vi "LDA Control.vi"() -> (1 "Error":errorcluster)   [LabVIEW 2022 SP3]
uses:
  File/Setup_Filetype.ctl
  Globals/LDA_global.vi
panel:
  out "Allowable":bool[](array[boolean])=[TRUE, TRUE, FALSE, FALSE, FALSE, TRUE, FALSE, FALSE, FALSE, FALSE, FALSE, FALSE]
  in  "Mode":i32(listbox)
  out "BSA IP Number":string
  out "Setup String":string
  out "Setup Filename":string
  out "reference out":refnum<k7>
  in  "SysMon":refnum<k7>(container)
  in  "Set Power (mW)":dbl=150.0
  in  "Laser":i32[](listbox)
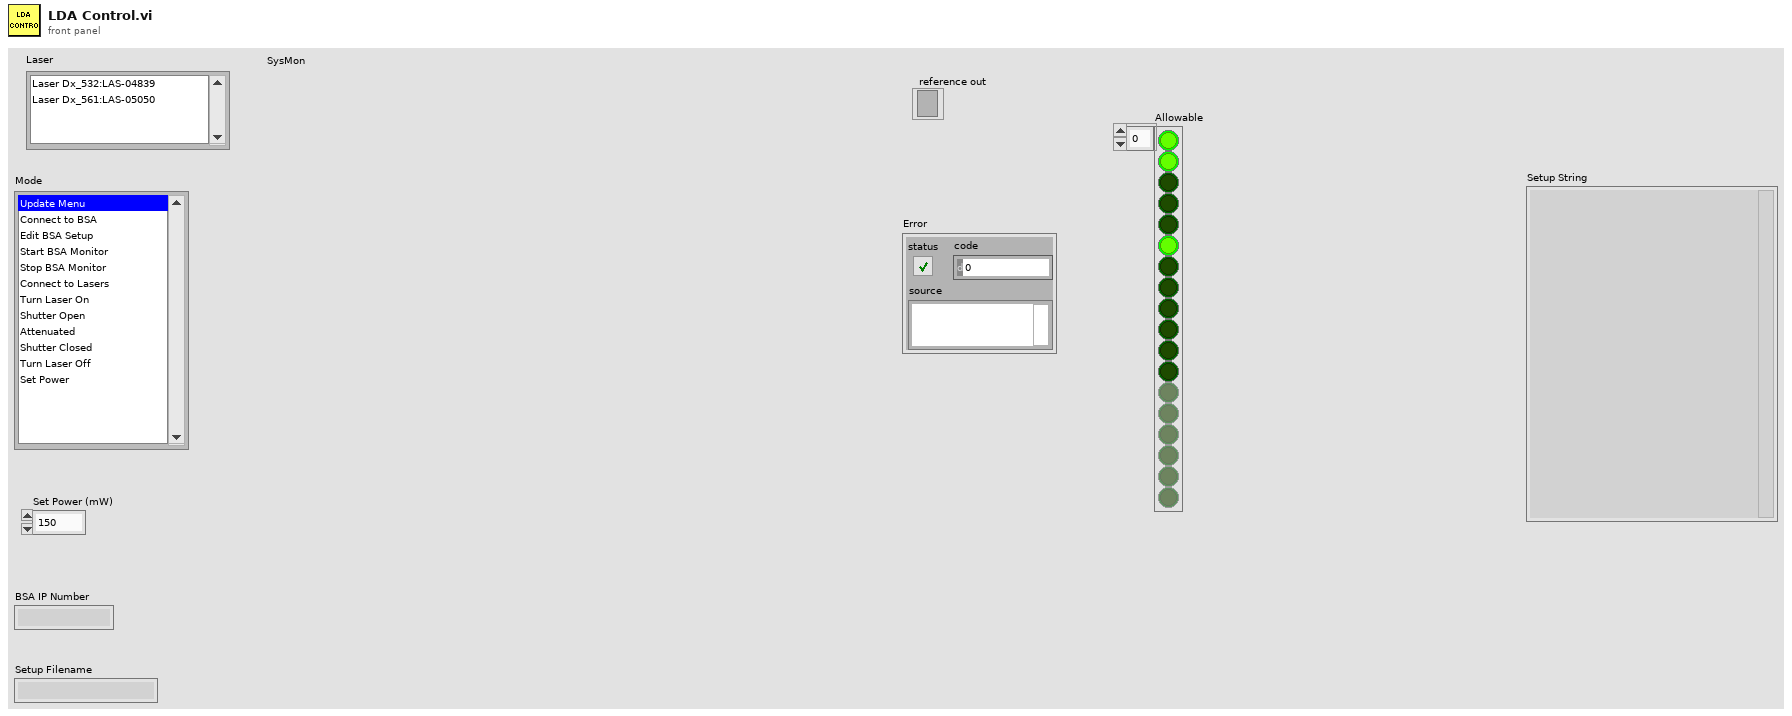
[diagram p1: front panel]
types:
  T1 = enum16{"Zero or one", "One", "Zero or more", "One or more"}
  T2 = typedef "Setup_Filetype.ctl" = enum16{"Measurement Setups", "Calibration Setups", "General", "Results File Plotter Setups", "Speed Calib Tweaks"}
  T3 = typedef "LDA_Channel.ctl" = cluster{"Wavelength (nm)":dbl, "Vel Comp":string, "Max Velocity":dbl, "Min Velocity":dbl, "Max Record length":u16, "Signal gain (dB)":i16, "High voltage":i16, "Optics Conversion Factor":dbl, "Min Record length":u16, "Multiply Velocity by -1":bool, "Signal to Noise Ratio":string, "Validation Ratio":string, "Probe":string, "Laser":string, "BSA":string, "Lense":string, "Beam Separation (mm)":dbl, "Focal Length (mm)":dbl, "COLOUR":u32, "BSA IP":string, "Velocity Range (m/s)":dbl, "Centre Velocity (m/s)":dbl, "Unshifted mW":dbl, "Shifted mW":dbl, "Bandwidth Hz":dbl, "Req Sampling Rate Hz":dbl, "Ch":i32, "CenterFreq Hz":dbl, "Laser IP":string, "Sync Delay (s)":dbl}
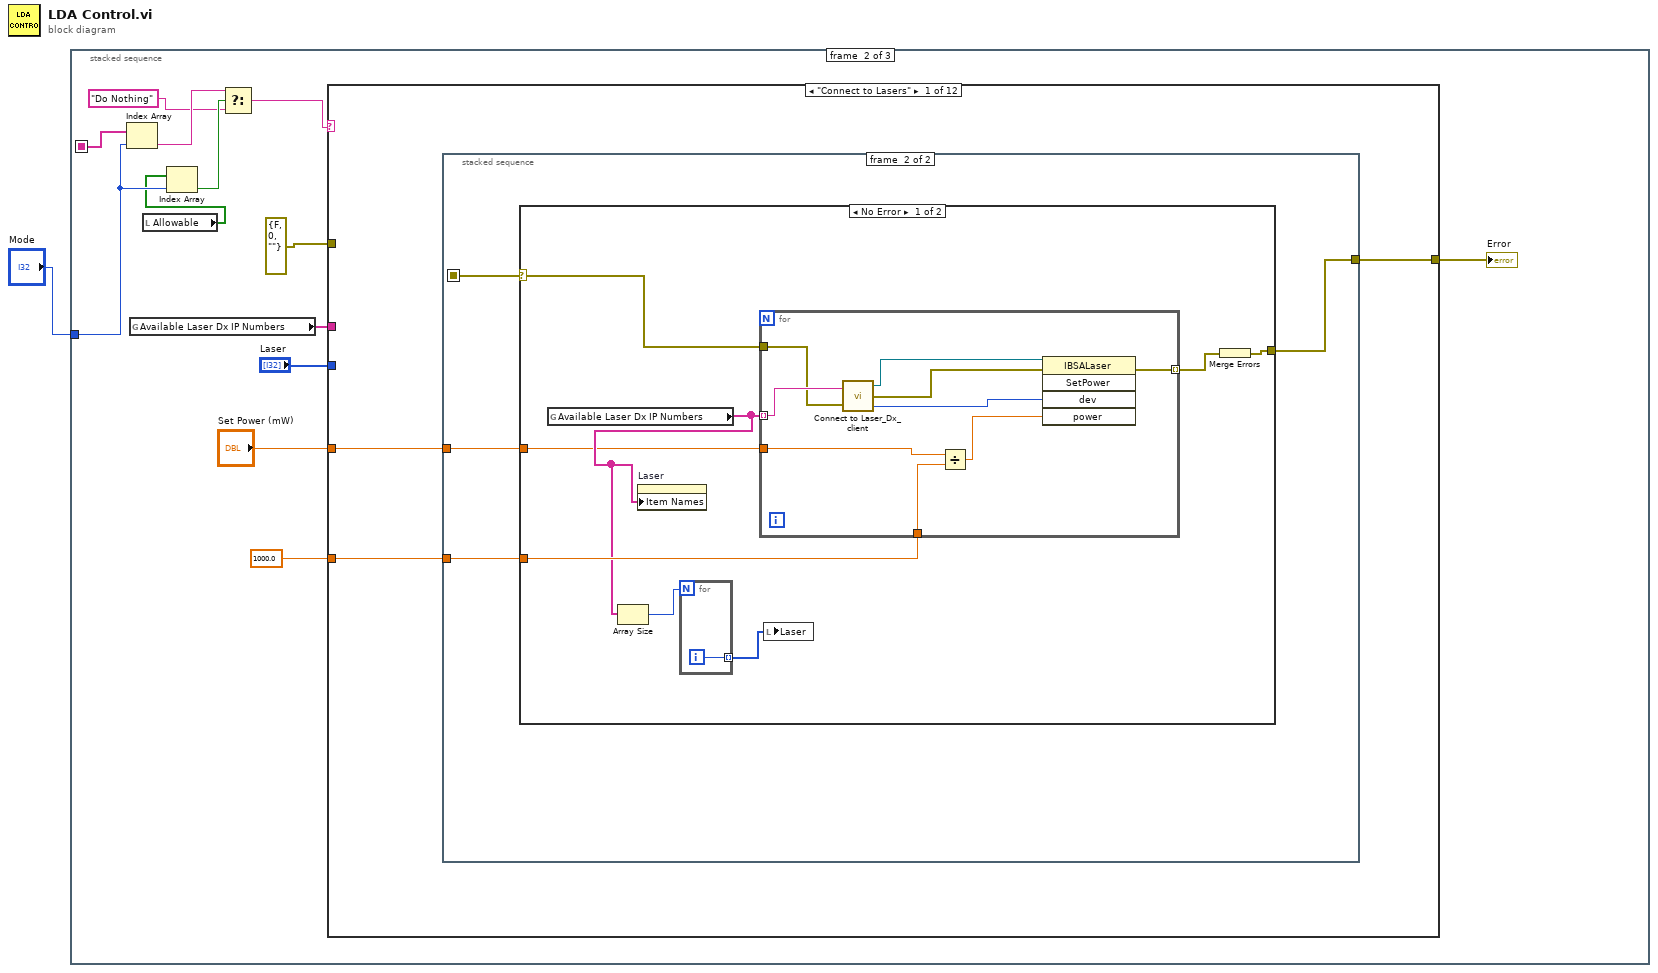
[diagram p0: block diagram]
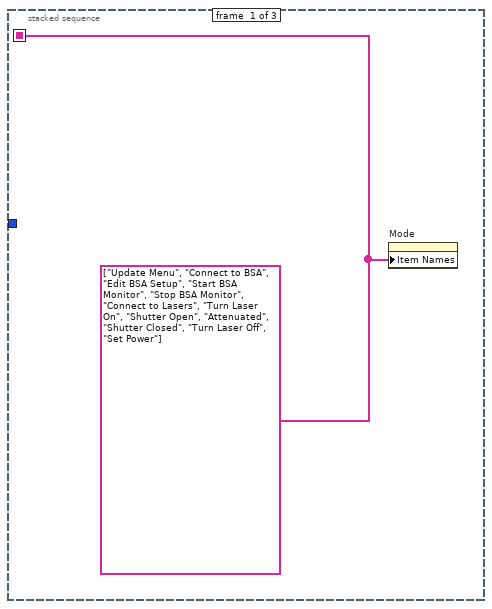
[diagram p2: hidden frame]
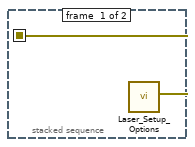
[diagram p3: hidden frame]
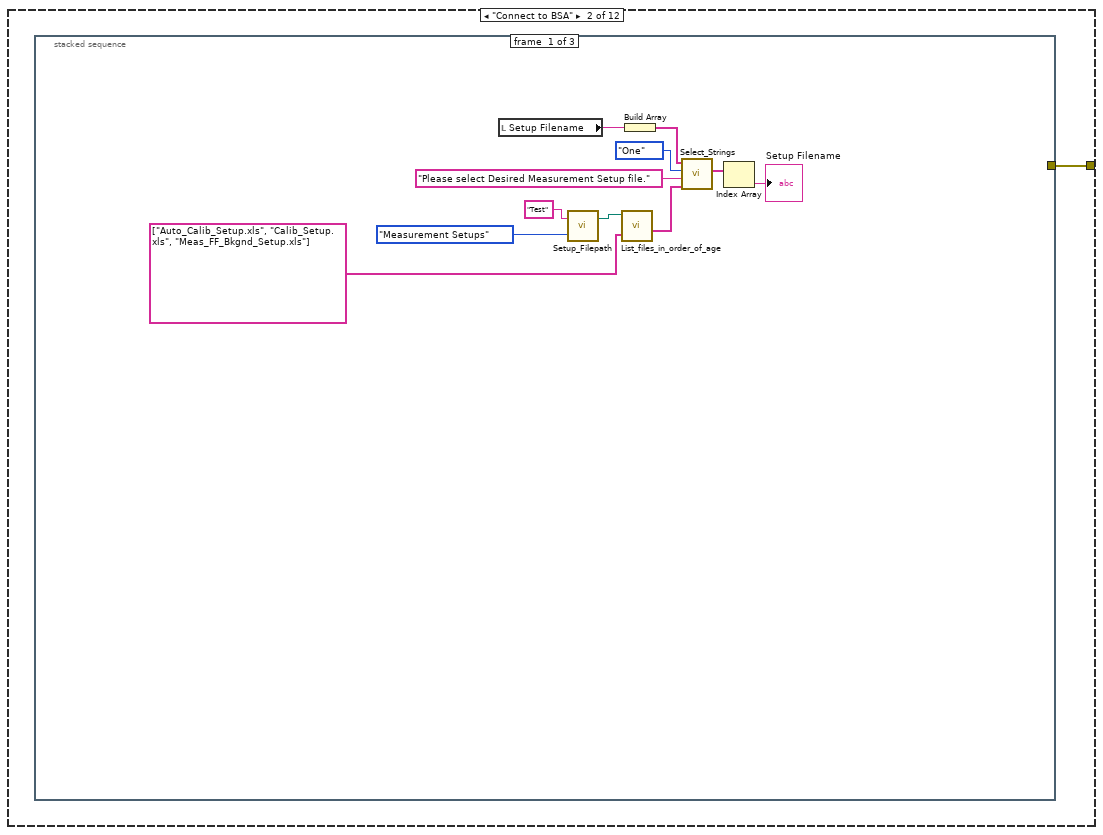
[diagram p5: hidden frame]
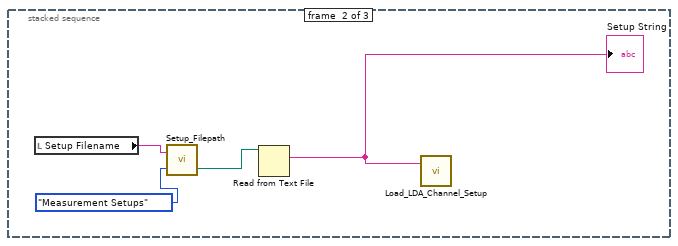
[diagram p6: hidden frame]
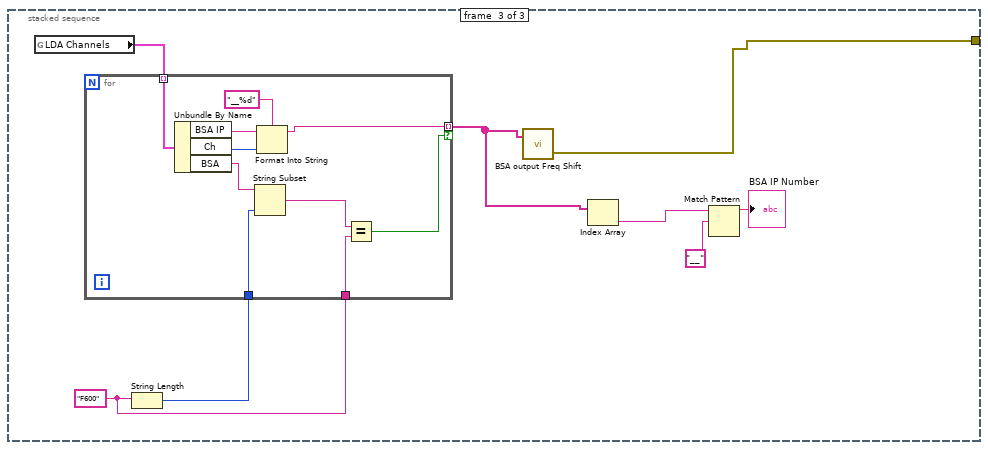
[diagram p7: hidden frame]
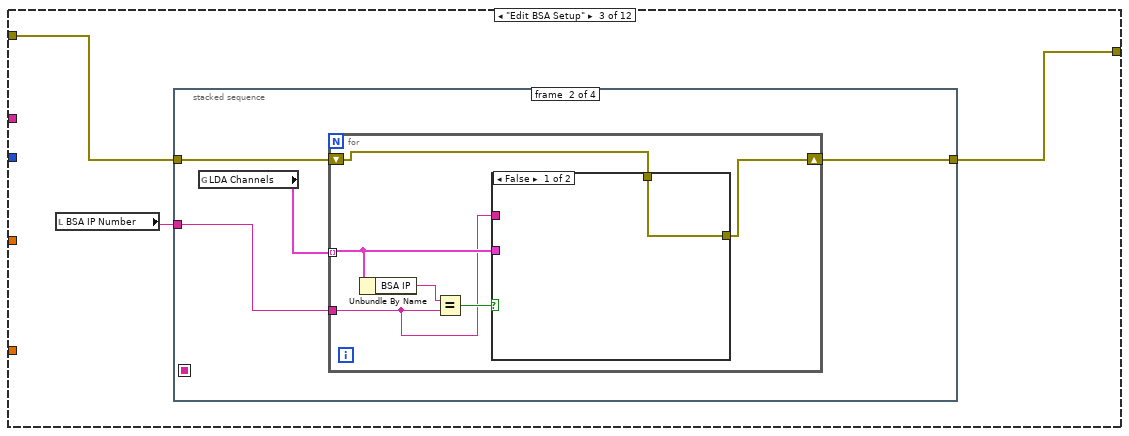
[diagram p8: hidden frame]
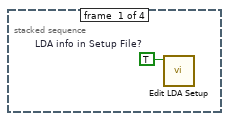
[diagram p9: hidden frame]
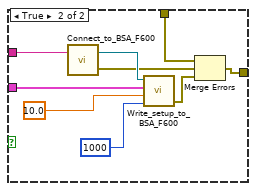
[diagram p10: hidden frame]
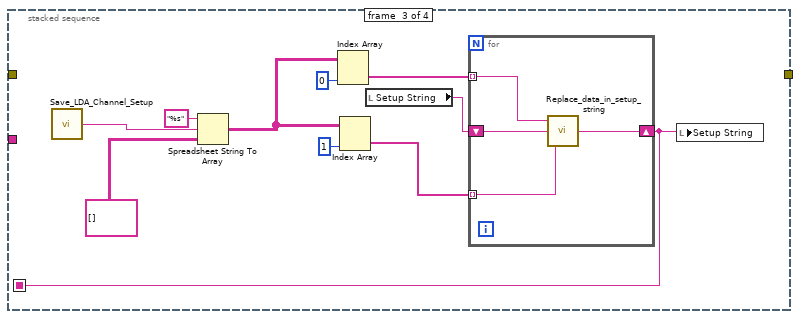
[diagram p11: hidden frame]
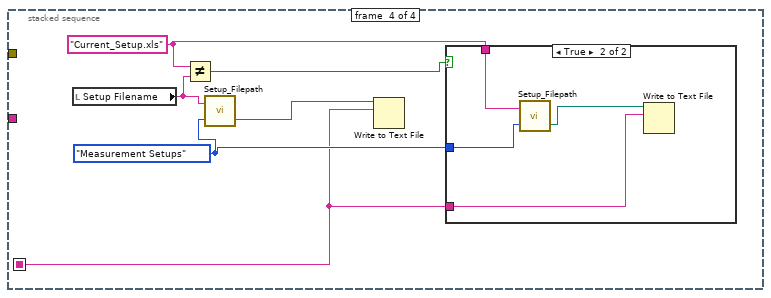
[diagram p12: hidden frame]
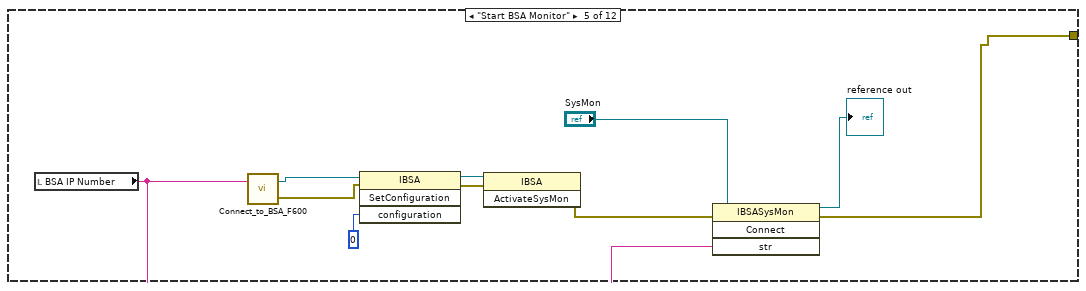
[diagram p15: hidden frame]
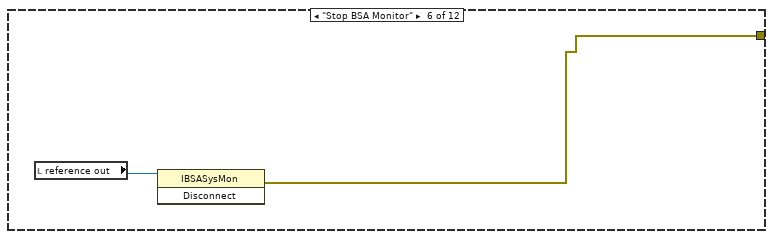
[diagram p16: hidden frame]
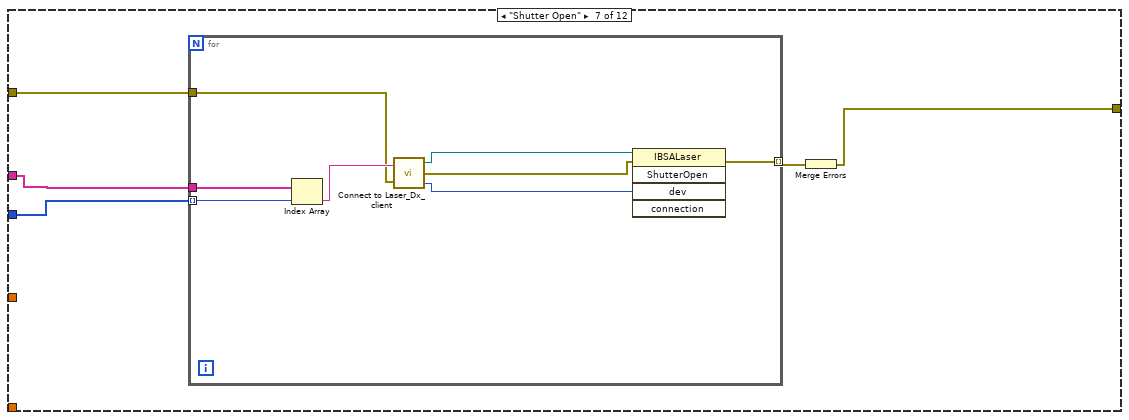
[diagram p17: hidden frame]
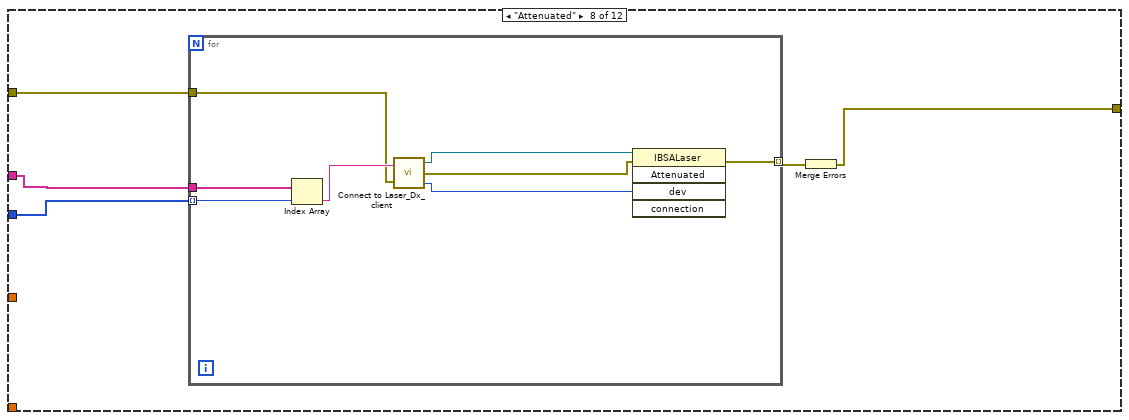
[diagram p18: hidden frame]
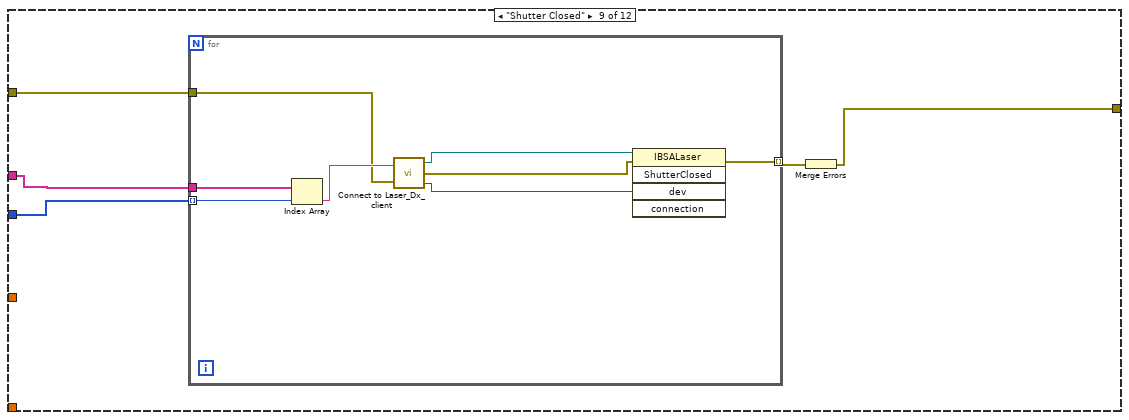
[diagram p19: hidden frame]
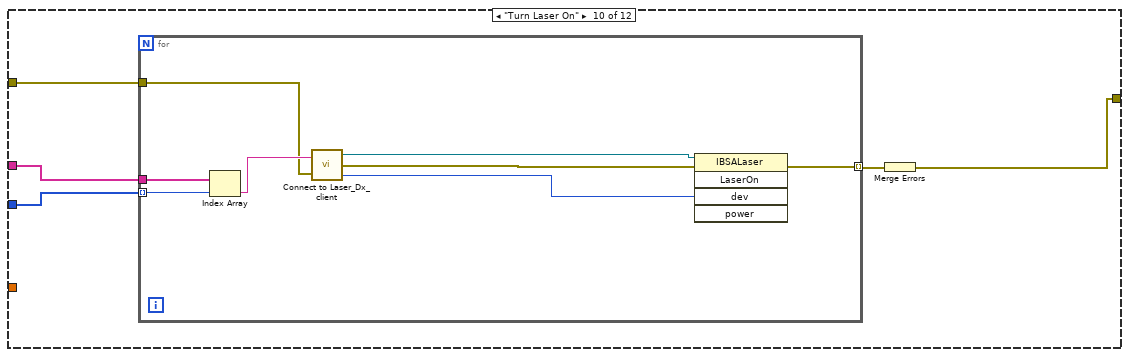
[diagram p20: hidden frame]
diagram:
  n1 = stacked-sequence {
    seq-local: [w2 _ _] -> [_ w11 _]
    tunnel: "Mode" -> [_ w8 _]
    frame #0 {
      w2 = string[] ["Update Menu", "Connect to BSA", "Edit BSA Setup", "Start BSA Monitor", "Stop BSA Monitor", "Connect to Lasers", "Turn Laser On", "Shutter Open", "Attenuated", "Shutter Closed", "Turn Laser Off", "Set Power"] ("Item Names")
      n2 = property on="Mode" class="LstBox (strict)"("Item Names"=w2) -> ()  [unwired: 2 in, 2 out]
    }
    frame #1 {
      n3 = Index Array(array=w11, index=w8) -> (element=w5:string)
      n4 = global read "LDA_global.vi" "Available Laser Dx IP Numbers"() -> (w13:string[])
      n5 = local read "Allowable"() -> (w7:bool[])
      n6 = Index Array(array=w7, index=w8) -> (element=w6:bool)
      n7 = Select(t=w5, s=w6, f="Do Nothing" ("t")) -> (s? t:f=w10:string)
      n8 = case shown="\"Connect to Lasers\"" w10 {
        tunnel: [w17 w43 w78 w125 w126 w136 w139 w152 w165 w178 w191 w205] -> w12
        tunnel: 1000.0 ("y") -> [w18 _ _ _ _ _ _ _ _ _ _ w209]
        tunnel: "Laser" -> [_ _ _ _ _ _ w141 w154 w167 w180 w193 w207]
        tunnel: w13 -> [_ _ _ _ _ _ w142 w155 w168 w181 w194 w208]
        tunnel: errorcluster {"status"=FALSE, "code"=0, "source"=""} ("error IO") -> [_ _ w77 w125 _ _ w138 w151 w164 w177 w190 w204]
        tunnel: "Set Power (mW)" -> [w16 _ _ _ _ _ _ _ _ _ _ w203]
        frame "Connect to Lasers" {
          n9 = stacked-sequence {
            seq-local: [w19 _] -> [_ w21]
            tunnel: w18 -> [_ w23]
            tunnel: [_ w22] -> w17
            tunnel: w16 -> [_ w20]
            frame #0 {
              n10 = call "Laser_Setup_Options.vi"() -> ("error out"=w19:errorcluster)  [unwired: 5 in, 3 out]
            }
            frame #1 {
              n11 = case shown="No Error" w21 {
                selector: w21 -> [w30 w42]
                tunnel: w23 -> [w31 _]
                tunnel: [w28 w42] -> w22
                tunnel: w20 -> [w24 _]
                frame No Error {
                  n12 = global read "LDA_global.vi" "Available Laser Dx IP Numbers"() -> (w27:string[])
                  n13 = Array Size(array=w27) -> (size(s)=w25:i32)
                  n14 = property on="Laser" class="LstBox (strict)"("Item Names"=w27) -> ()  [unwired: 2 in, 2 out]
                  n15 = for {
                    N: w25 -> [_]
                    tunnel: [w32] -> w26 mode=indexing
                    i -> [w32]
                  }
                  n16 = for {
                    tunnel: w27 -> [w36] mode=indexing
                    tunnel: w31 -> [w41]
                    tunnel: w30 -> [w35]
                    tunnel: [w34] -> w29 mode=indexing
                    tunnel: w24 -> [w33]
                    n17 = call "Connect to Laser_Dx_client.vi"("Laser IP Number"=w36, "error in (no error)"=w35) -> ("Laser_Dx"=w39:refnum<k7>, "error out"=w38:errorcluster, "Channel"=w37:i64)
                    n18 = Divide(x=w33, y=w41) -> (x/y=w40:dbl)
                    n19 = invoke class="IBSALaser" method="SetPower"(reference=w39, error in=w38, "dev"=w37, "power"=w40) -> (error out=w34:errorcluster)  [unwired: 1 in, 4 out]
                  }
                  n20 = local write "Laser"(w26) -> ()
                  n21 = Merge Errors(w29) -> (w28:errorcluster)
                }
                frame Error {
                }
              }
            }
          }
        }
        frame "Connect to BSA" {
          n22 = stacked-sequence {
            tunnel: [_ _ w65] -> w43
            frame #0 {
              n23 = local read "Setup Filename"() -> (w52:string)
              n24 = call "Setup_Filepath.vi"("Setup File Type"=Setup_Filetype."Measurement Setups", "Filename in"="Test") -> ("Directory"=w49:path)  [unwired: 1 out]
              n25 = call "List_files_in_order_of_age.vi"("Files to Hide"=string[] ["Auto_Calib_Setup.xls", "Calib_Setup.xls", "Meas_FF_Bkgnd_Setup.xls"] ("file names"), "Folder"=w49) -> ("file names"=w50:string[])  [unwired: 9 in]
              n26 = Build Array(w52) -> (w53:string[])
              n27 = call "Select_Strings.vi"("Available Ch names"=w50, "Message"="Please select Desired Measurement Setup file.", "Selector mode"=T1."One", "Desired Ch names (in)"=w53) -> ("Selected Channel Names"=w51:string[])  [unwired: 2 in, 2 out]
              n28 = Index Array(array=w51) -> (element=→"Setup Filename":string)  [unwired: 1 in]
            }
            frame #1 {
              n29 = local read "Setup Filename"() -> (w58:string)
              n30 = call "Setup_Filepath.vi"("Setup File Type"=Setup_Filetype."Measurement Setups", "Filename in"=w58) -> ("Filename Out"=w56:path)  [unwired: 1 out]
              n31 = Read from Text File(file (use dialog)=w56) -> (text=w57:string)  [unwired: 3 in, 3 out]
              "Setup String" <- w57
              n32 = call "Load_LDA_Channel_Setup.vi"("Setup file string"=w57) -> ()  [unwired: 2 in]
            }
            frame #2 {
              w59 = "F600"
              n33 = global read "LDA_global.vi" "LDA Channels"() -> (w66:T3[])
              n34 = String Length(string=w59) -> (length=w60:i32)
              n35 = for {
                tunnel: [w72] -> w62 mode=indexing if=w67
                tunnel: w66 -> [w76] mode=indexing
                tunnel: w60 -> [w70]
                tunnel: w59 -> [w68]
                n36 = Unbundle By Name(w76) -> ("BSA IP"=w74:string, "Ch"=w75:i32, "BSA"=w71:string)
                n37 = String Subset(string=w71, length (rest)=w70) -> (substring=w69:string)  [unwired: 1 in]
                n38 = Format Into String(format string="__%d", initial string=w74, w75) -> (resulting string=w72:string)  [unwired: 1 in, 1 out]
                n39 = Equal?(x=w69, y=w68) -> (x = y?=w67:bool)
              }
              n40 = call "BSA output Freq Shift.vi"("BSAIP__ChNum"=w62) -> ("BSA Error"=w65:errorcluster)  [unwired: 2 in]
              n41 = Index Array(array=w62) -> (element=w64:string)  [unwired: 1 in]
              n42 = Match Pattern(string=w64, regular expression="__" ("string")) -> (before substring=→"BSA IP Number":string)  [unwired: 1 in, 3 out]
            }
          }
        }
        frame "Edit BSA Setup" {
          n43 = local read "BSA IP Number"() -> (w79:string)
          n44 = stacked-sequence {
            seq-local: [_ _ w101 _] -> [_ _ _ w115]
            tunnel: w79 -> [_ w83 _ _]
            tunnel: [_ w82 _ _] -> w78
            tunnel: w77 -> [_ w81 _ _]
            frame #0 {
              w80 = TRUE  # LDA info in Setup File?
              n45 = call "Edit LDA Setup.vi"("LDA info in Setup File?"=w80) -> ()  [unwired: 11 in]
            }
            frame #1 {
              n46 = global read "LDA_global.vi" "LDA Channels"() -> (w84:T3[])
              n47 = for {
                tunnel: w84 -> [w90] mode=indexing
                tunnel: w83 -> [w87]
                shift-right: [w85] -> w82
                shift-left: w81 -> [w86]
                n48 = Unbundle By Name(w90) -> ("BSA IP"=w89:string)
                n49 = Equal?(x=w89, y=w87) -> (x = y?=w88:bool)
                n50 = case shown="False" w88 {
                  tunnel: w90 -> [_ w98]
                  tunnel: w87 -> [_ w97]
                  tunnel: [w91 w93] -> w85
                  tunnel: w86 -> [w91 w92]
                  frame False {
                  }
                  frame True {
                    n51 = call "Connect_to_BSA_F600.vi"("BSA IP Number"=w97) -> ("error out"=w94:errorcluster, "F600"=w96:refnum<k7>)  [unwired: 1 in]
                    n52 = call "Write_setup_to_BSA_F600.vi"("No Of Samples"=1000, "Time (s)"=sgl 10.0, "BSA Setup In"=w98, "BSACtrl.IBSA F600"=w96) -> ("error out"=w95:errorcluster)  [unwired: 2 out]
                    n53 = Merge Errors(w92, w94, w95) -> (w93:errorcluster)
                  }
                }
              }
            }
            frame #2 {
              n54 = call "Save_LDA_Channel_Setup.vi"() -> ("Setup file string"=w110:string)  [unwired: 1 in]
              n55 = Spreadsheet String To Array(format string="%s", spreadsheet string=w110, array type (2D Dbl)=string[][] []) -> (array=w109:string[][])  [unwired: 1 in]
              n56 = Index Array(array=w109, index (col)=0 ("disabled index (col)")) -> (element=w108:string[])  [unwired: 1 in]
              n57 = Index Array(array=w109, index (col)=1 ("disabled index (col)")) -> (element=w107:string[])  [unwired: 1 in]
              n58 = local read "Setup String"() -> (w106:string)
              n59 = for {
                tunnel: w108 -> [w114] mode=indexing
                tunnel: w107 -> [w112] mode=indexing
                shift-right: [w111] -> w101
                shift-left: w106 -> [w113]
                n60 = call "Replace_data_in_setup_string.vi"("New data string"=w112, "Input string"=w113, "Variable name"=w114) -> ("Appended string"=w111:string)
              }
              n61 = local write "Setup String"(w101) -> ()
            }
            frame #3 {
              w117 = "Current_Setup.xls"
              w116 = Setup_Filetype."Measurement Setups" ("Setup File Type")
              n62 = local read "Setup Filename"() -> (w119:string)
              n63 = Not Equal?(x=w117, y=w119) -> (x != y?=w118:bool)
              n64 = call "Setup_Filepath.vi"("Setup File Type"=w116, "Filename in"=w119) -> ("Filename Out"=w120:path)  [unwired: 1 out]
              n65 = Write to Text File(file (use dialog)=w120, text=w115) -> ()  [unwired: 2 in, 3 out]
              n66 = case shown="True" w118 {
                tunnel: w117 -> [_ w124]
                tunnel: w116 -> [_ w123]
                tunnel: w115 -> [_ w122]
                frame False {
                }
                frame True {
                  n67 = call "Setup_Filepath.vi"("Setup File Type"=w123, "Filename in"=w124) -> ("Filename Out"=w121:path)  [unwired: 1 out]
                  n68 = Write to Text File(file (use dialog)=w121, text=w122) -> ()  [unwired: 2 in, 3 out]
                }
              }
            }
          }
        }
        frame "Do Nothing", Default {
        }
        frame "Start BSA Monitor" {
          n69 = local read "BSA IP Number"() -> (w127:string)
          n70 = call "Connect_to_BSA_F600.vi"("BSA IP Number"=w127) -> ("error out"=w135:errorcluster, "F600"=w134:refnum<k7>)  [unwired: 1 in]
          n71 = invoke class="IBSA" method="SetConfiguration"(reference=w134, error in=w135, "configuration"=0 ("config")) -> (reference out=w130:refnum<k7>, error out=w129:errorcluster)  [unwired: 1 in, 2 out]
          n72 = invoke class="IBSA" method="ActivateSysMon"(reference=w130, error in=w129) -> (error out=w131:errorcluster)  [unwired: 1 in, 2 out]
          n73 = invoke class="IBSASysMon" method="Connect"(reference="SysMon", error in=w131, "str"=w127) -> (reference out=→"reference out":refnum<k7>, error out=w126:errorcluster)  [unwired: 1 in, 2 out]
        }
        frame "Stop BSA Monitor" {
          n74 = local read "reference out"() -> (w137:refnum<k7>)
          n75 = invoke class="IBSASysMon" method="Disconnect"(reference=w137) -> (error out=w136:errorcluster)  [unwired: 2 in, 2 out]
        }
        frame "Shutter Open" {
          n76 = for {
            tunnel: [w150] -> w140 mode=indexing
            tunnel: w142 -> [w148]
            tunnel: w141 -> [w147] mode=indexing
            tunnel: w138 -> [w143]
            n77 = Index Array(array=w148, index=w147) -> (element=w149:string)
            n78 = call "Connect to Laser_Dx_client.vi"("Laser IP Number"=w149, "error in (no error)"=w143) -> ("Laser_Dx"=w146:refnum<k7>, "error out"=w145:errorcluster, "Channel"=w144:i64)
            n79 = invoke class="IBSALaser" method="ShutterOpen"(reference=w146, error in=w145, "dev"=w144) -> (error out=w150:errorcluster)  [unwired: 2 in, 4 out]
          }
          n80 = Merge Errors(w140) -> (w139:errorcluster)
        }
        frame "Attenuated" {
          n81 = for {
            tunnel: [w163] -> w153 mode=indexing
            tunnel: w155 -> [w161]
            tunnel: w154 -> [w160] mode=indexing
            tunnel: w151 -> [w156]
            n82 = Index Array(array=w161, index=w160) -> (element=w162:string)
            n83 = call "Connect to Laser_Dx_client.vi"("Laser IP Number"=w162, "error in (no error)"=w156) -> ("Laser_Dx"=w159:refnum<k7>, "error out"=w158:errorcluster, "Channel"=w157:i64)
            n84 = invoke class="IBSALaser" method="Attenuated"(reference=w159, error in=w158, "dev"=w157) -> (error out=w163:errorcluster)  [unwired: 2 in, 4 out]
          }
          n85 = Merge Errors(w153) -> (w152:errorcluster)
        }
        frame "Shutter Closed" {
          n86 = for {
            tunnel: [w176] -> w166 mode=indexing
            tunnel: w168 -> [w174]
            tunnel: w167 -> [w173] mode=indexing
            tunnel: w164 -> [w169]
            n87 = Index Array(array=w174, index=w173) -> (element=w175:string)
            n88 = call "Connect to Laser_Dx_client.vi"("Laser IP Number"=w175, "error in (no error)"=w169) -> ("Laser_Dx"=w172:refnum<k7>, "error out"=w171:errorcluster, "Channel"=w170:i64)
            n89 = invoke class="IBSALaser" method="ShutterClosed"(reference=w172, error in=w171, "dev"=w170) -> (error out=w176:errorcluster)  [unwired: 2 in, 4 out]
          }
          n90 = Merge Errors(w166) -> (w165:errorcluster)
        }
        frame "Turn Laser On" {
          n91 = for {
            tunnel: w181 -> [w189]
            tunnel: w180 -> [w188] mode=indexing
            tunnel: [w183] -> w179 mode=indexing
            tunnel: w177 -> [w182]
            n92 = Index Array(array=w189, index=w188) -> (element=w187:string)
            n93 = call "Connect to Laser_Dx_client.vi"("Laser IP Number"=w187, "error in (no error)"=w182) -> ("Laser_Dx"=w186:refnum<k7>, "error out"=w185:errorcluster, "Channel"=w184:i64)
            n94 = invoke class="IBSALaser" method="LaserOn"(reference=w186, error in=w185, "dev"=w184) -> (error out=w183:errorcluster)  [unwired: 2 in, 4 out]
          }
          n95 = Merge Errors(w179) -> (w178:errorcluster)
        }
        frame "Turn Laser Off" {
          n96 = for {
            tunnel: [w202] -> w192 mode=indexing
            tunnel: w194 -> [w200]
            tunnel: w193 -> [w199] mode=indexing
            tunnel: w190 -> [w195]
            n97 = Index Array(array=w200, index=w199) -> (element=w201:string)
            n98 = call "Connect to Laser_Dx_client.vi"("Laser IP Number"=w201, "error in (no error)"=w195) -> ("Laser_Dx"=w198:refnum<k7>, "error out"=w197:errorcluster, "Channel"=w196:i64)
            n99 = invoke class="IBSALaser" method="LaserOff"(reference=w198, error in=w197, "dev"=w196) -> (error out=w202:errorcluster)  [unwired: 1 in, 3 out]
          }
          n100 = Merge Errors(w192) -> (w191:errorcluster)
        }
        frame "Set Power" {
          n101 = for {
            tunnel: [w220] -> w206 mode=indexing
            tunnel: w209 -> [w218]
            tunnel: w208 -> [w216]
            tunnel: w207 -> [w212] mode=indexing
            tunnel: w204 -> [w211]
            tunnel: w203 -> [w210]
            n102 = Index Array(array=w216, index=w212) -> (element=w217:string)
            n103 = call "Connect to Laser_Dx_client.vi"("Laser IP Number"=w217, "error in (no error)"=w211) -> ("Laser_Dx"=w215:refnum<k7>, "error out"=w214:errorcluster, "Channel"=w213:i64)
            n104 = Divide(x=w210, y=w218) -> (x/y=w219:dbl)
            n105 = invoke class="IBSALaser" method="SetPower"(reference=w215, error in=w214, "dev"=w213, "power"=w219) -> (error out=w220:errorcluster)  [unwired: 1 in, 4 out]
          }
          n106 = Merge Errors(w206) -> (w205:errorcluster)
        }
      }
      "Error" <- w12
    }
    frame #2 {
      w223 = FALSE
      n107 = global read "LDA_global.vi" "Connected Laser Dx IPs"() -> (w234:string[])
      n108 = Array Size(array=w234) -> (size(s)=w233:i32)
      n109 = Equal To 0?(x=w233) -> (x = 0?=w221:bool)
      n110 = global read "LDA_global.vi" "Connected BSA IPs"() -> (w226:string[])
      n111 = case shown="False" w221 {
        tunnel: [w238 w239] -> w222
        frame False {
          n112 = global read "LDA_global.vi" "Available Laser Dx names"() -> (w238:string[])
        }
        frame True {
          w239 = string[] [] ("Available Laser Dx names")
          n113 = global write "LDA_global.vi" "Available Laser Dx IP Numbers"(w239) -> ()
          n114 = global write "LDA_global.vi" "Available Laser Dx names"(w239) -> ()
        }
      }
      n115 = Array Size(array=w226) -> (size(s)=w225:i32)
      n116 = Equal To 0?(x=w225) -> (x = 0?=w224:bool)
      n117 = Initialize Array(w224, 3 ("dimension size")) -> (w236:bool[])
      n118 = Build Array (concatenate)(w223, w223, w236) -> (w229:bool[])
      n119 = Initialize Array(w221, 6 ("dimension size")) -> (w231:bool[])
      n120 = Build Array (concatenate)(FALSE, w231) -> (w230:bool[])
      n121 = Build Array (concatenate)(w229, w230) -> (w228:bool[])
      n122 = property on="Laser" class="LstBox (strict)"("Item Names"=w222) -> ()  [unwired: 2 in, 2 out]
      n123 = Not(x=w228) -> (.not. x?=→"Allowable":bool[])
      n124 = for {
        tunnel: w228 -> [w243] mode=indexing
        i -> [w244]
        n125 = Select(t=u32 13816530 ("Active Row:Cell Font:Color"), s=w243, f=u32 0 ("Active Row:Cell Font:Color")) -> (s? t:f=w240:u32)
        n126 = property on="Mode" class="LstBox (strict)"("Active Row"=w244, "CellFontStrike"=w243, "CellFontColor"=w240) -> ()  [unwired: 2 in, 2 out]
      }
    }
  }
